vi "Get Destination IP and ID.vi"(8 "error in (no error)":errorcluster, 11 "TCP Writer in":refnum<class "TCP Writer.lvclass">) -> (0 "error out":errorcluster, 3 "TCP Writer out":refnum<class "TCP Writer.lvclass">)   [LabVIEW 2026, in "TALOS.lvlib" / "TCP Writer.lvlib" / "TCP Writer.lvclass"]
uses:
  TCP Writer.lvclass
  C:/LabVIEW Code/TALOS/talos/Ancestor/Ancestor/Ancestor.lvclass
  Ancestor/Ancestor/Ancestor.lvclass/Ancestor.ctl
  <vilib>/Utility/error.llb/Trim Whitespace (string).vi
  Ancestor/Ancestor/Read ID.vi
  <vilib>/Utility/error.llb/Trim Whitespace One-Sided.vi
  Support VIs/Circus Config Param - Core.vi
  Support VIs/Generate Error.vi
  Support VIs/Circus Root Path.vi
  Support VIs/TALOS Config Param.vi
  FGV/Error Memory/Get Error Description.vi
  Support VIs/Get PC name.vi
  Support VIs/Get Class Name.vi
  <vilib>/Utility/error.llb/Clear Errors.vi
  FGV/Error Memory/Error Memory Core.vi
  <vilib>/AdvancedString/Delimited String to 1D String Array.vi
  <vilib>/AdvancedString/Delimited String to 1D String Array (string).vi
  FGV/Error Memory/Error Crt Lvl checker.vi
  FGV/Error Memory/Error Memory Core.vi/40c8088d-b597-4017-91af-faa98e00292e.vi
  FGV/Error Memory/Error Memory Core.vi/d4a3ab98-063c-4e44-b43d-fbdcfe6c2be2.vi
  Support VIs/Global Memory.vi
  <vilib>/Utility/LVClass/Get LV Class Name.vi
  Support VIs/Is in Packed Library.vi
  Support VIs/TALOS Root path.vi
  Support VIs/Read CSV worksheet.vi
  Support VIs/Global Constants.vi
  <vilib>/Utility/error.llb/General Error Handler.vi
  <vilib>/Utility/config.llb/Open Config Data.vi
  <vilib>/Utility/config.llb/Get Section Names.vi
  <vilib>/Utility/config.llb/Get Key Names.vi
  <vilib>/Utility/config.llb/Read Key.vi
  <vilib>/Utility/config.llb/Read Key (String).vi
  <vilib>/Utility/config.llb/Close Config Data.vi
  Guardian/Guardian/Extract list from Project INI file entry.vi
  Ancestor/Ancestor/Ancestor.lvclass
  <vilib>/Comparison/Equal/Equal Functor/Equal Functor.lvclass
  TALOS.lvlib
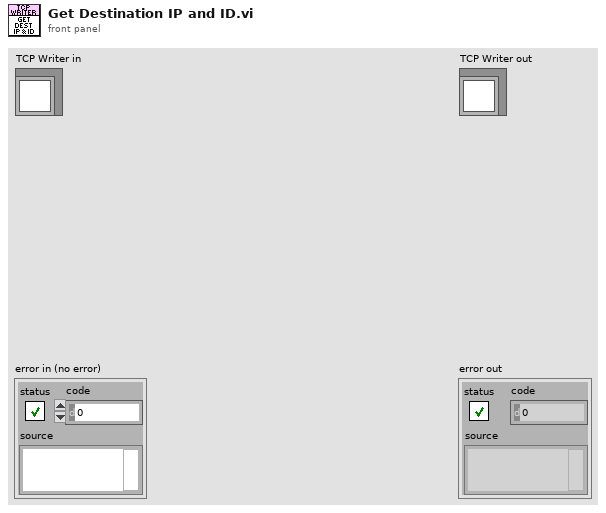
[diagram p1: front panel]
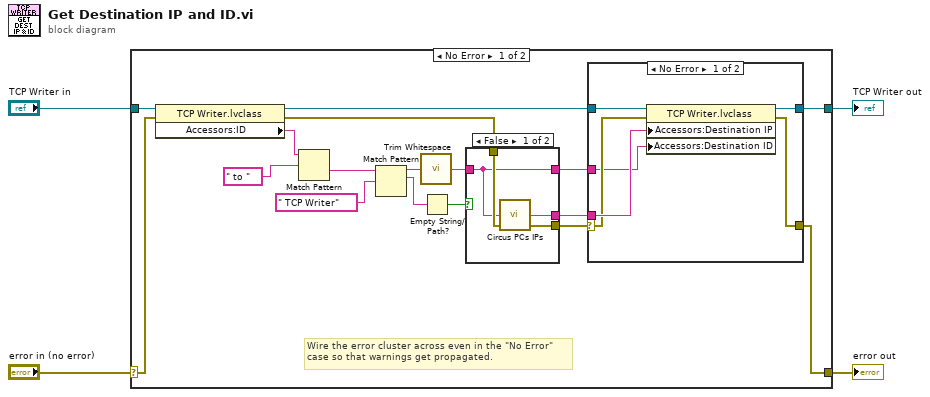
[diagram p0: block diagram]
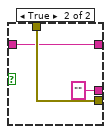
[diagram p3: hidden frame]
diagram:
  n1 = case shown="No Error" "error in (no error)" {
    selector: "error in (no error)" -> [w7 w38]
    tunnel: [w8 w38] -> w3
    tunnel: [w13 w37] -> w1
    tunnel: "TCP Writer in" -> [w21 w37]
    frame No Error {
      # "Wire the error cluster across even in the \"No Error\"\ncase so that warnings get propagated."
      n2 = property class="TCP Writer.lvclass"(reference=w21, error in=w7) -> (reference out=w20:refnum<class "TCP Writer.lvclass">, error out=w6:errorcluster, "Accessors:ID"=w16:string)
      n3 = Match Pattern(string=w16, regular expression=" to ") -> (after substring=w17:string)  [unwired: 1 in, 3 out]
      n4 = Match Pattern(string=w17, regular expression=" TCP Writer") -> (before substring=w11:string, match substring=w14:string)  [unwired: 1 in, 2 out]
      n5 = call-poly <vilib>:"Trim Whitespace.vi"("string"=w11) -> ("trimmed string"=w10:string)  [unwired: 1 in]
      n6 = Empty String/Path?(string/path=w14) -> (empty?=w15:bool)
      n7 = case shown="False" w15 {
        tunnel: w10 -> [w30 w34]
        tunnel: [w33 "" ("IP")] -> w12
        tunnel: [w32 w35] -> w9
        tunnel: w6 -> [w31 w35]
        tunnel: [w30 w34] -> w5
        frame False {
          n8 = call "Circus PCs IPs.vi"("error in (no error)"=w31, "ID"=w30) -> ("error out"=w32:errorcluster, "IP"=w33:string)  [unwired: 2 in]
        }
        frame True {
        }
      }
      n9 = case shown="No Error" w9 {
        selector: w9 -> [w24 w28]
        tunnel: w20 -> [w27 w29]
        tunnel: [w26 w29] -> w13
        tunnel: w12 -> [w25 _]
        tunnel: [w23 w28] -> w8
        tunnel: w5 -> [w22 _]
        frame No Error {
          n10 = property class="TCP Writer.lvclass"(reference=w27, error in=w24, "Accessors:Destination IP"=w25, "Accessors:Destination ID"=w22) -> (reference out=w26:refnum<class "TCP Writer.lvclass">, error out=w23:errorcluster)
        }
        frame Error {
        }
      }
    }
    frame Error {
    }
  }
  "error out" <- w3
  "TCP Writer out" <- w1
